vi "Connect.vi"(8 "error in (no error)":errorcluster, 11 "NI Vision Camera Device in":refnum<class "NI Vision Camera Device.lvclass">) -> (0 "error out":errorcluster, 3 "NI Vision Camera Device out":refnum<class "NI Vision Camera Device.lvclass">)   [LabVIEW 2014, in "NI Vision Camera Device.lvclass"]
uses:
  NI Vision Camera Device.lvclass
  <vilib>/userdefined/High Color/IMAQdx.ctl
  NI Vision Camera Device.lvclass/NI Vision Camera Device.ctl
  <vilib>/vision/driver/NI_Vision_Acquisition_Software.lvlib
  <resource>/objmgr/imaqdx.rc
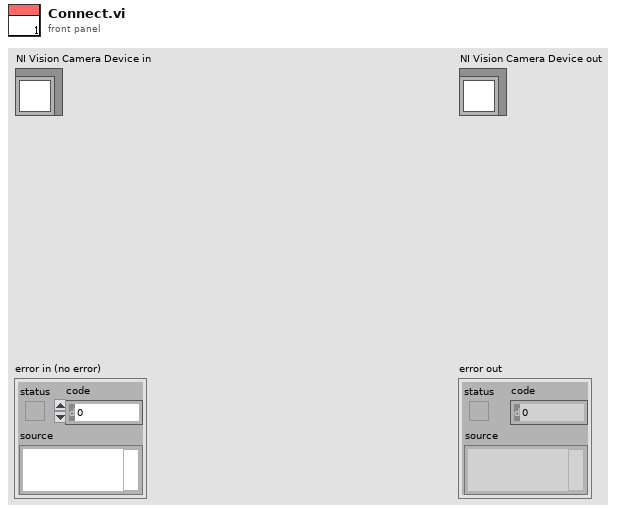
[diagram p1: front panel]
types:
  T1 = typedef "IMAQdx.ctl" = refnum<k21>
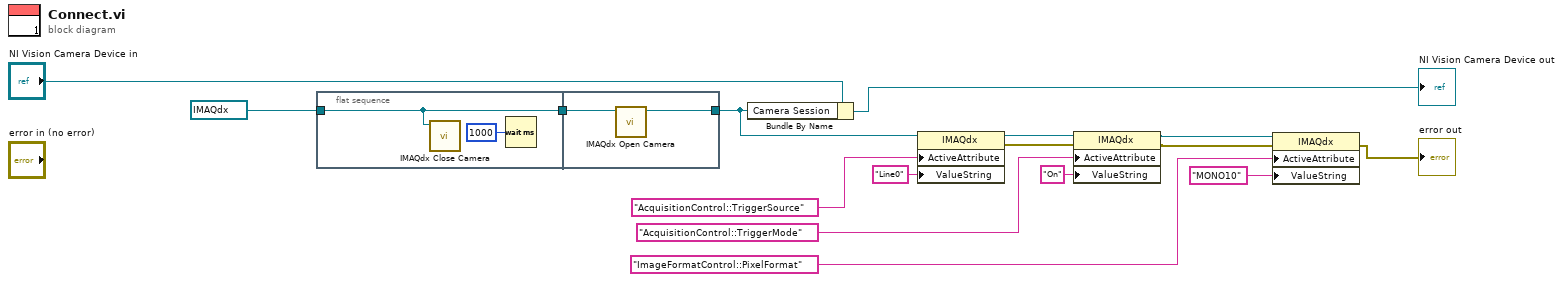
[diagram p0: block diagram]
diagram:
  n1 = flat-sequence {
    tunnel: T1 "cam0" ("Session In") -> [w18]
    tunnel: [w18] -> w1
    tunnel: [w19] -> w3
    tunnel: w1 -> [w20]
    frame #0 {
      n2 = call <vilib>:"IMAQdx Close Camera.vi"("Session In"=w18) -> ()  [unwired: 10 in, 1 out]
      n3 = Wait (ms)(milliseconds to wait=u32 1000) -> ()  [unwired: 1 out]
    }
    frame #1 {
      n4 = call <vilib>:"IMAQdx Open Camera.vi"("Session In"=w20) -> ("Session Out"=w19:T1)  [unwired: 9 in, 1 out]
    }
  }
  n5 = Bundle By Name(cluster="NI Vision Camera Device in", "Camera Session"=w3) -> (→"NI Vision Camera Device out":refnum<class "NI Vision Camera Device.lvclass">)
  n6 = property class="IMAQdx"(reference=w3, "ActiveAttribute"="AcquisitionControl::TriggerSource", "ValueString"="Line0") -> (reference out=w15:T1, error out=w14:errorcluster)  [unwired: 1 in]
  n7 = property class="IMAQdx"(reference=w15, error in=w14, "ActiveAttribute"="AcquisitionControl::TriggerMode", "ValueString"="On") -> (reference out=w7:T1, error out=w6:errorcluster)
  n8 = property class="IMAQdx"(reference=w7, error in=w6, "ActiveAttribute"="ImageFormatControl::PixelFormat", "ValueString"="MONO10") -> (error out=→"error out":errorcluster)  [unwired: 1 out]
